vi "fsk_test3_rx.vi"(0 "passband waveform (complex)":T1={"t0"=0.0, "dt"=1.0, "Y"=[]} {"Y" format="%.3f"; "dt" format="%^.2e"; "t0" format="%.4f"}, 1 "FSK system parameters":T2={"samples per symbol (16)"=16, "symbol map"=[], "symbol phase continuity"=enum."continuous"} {"symbol map" format="%.2f"}, 2 "VCO carrier frequency (Hz)":dbl, 3 "passband bandwidth (Hz)":dbl format="%.2p", 4 "reset? (F)":bool, 5 "error in (no error)":errorcluster, 6 "expected sync location (symbols)":i32=-1, 7 "pulse shaping filter coefficients":dbl[](array[numeric]) format="%.2f", 8 "sync location uncertainty (symbols)":i32=10, 9 "matched filter coefficients":dbl[](array[numeric]) format="%.2f", 11 "sync bits":i8[](array[numeric]), 13 "Key Bit Sequence":u32[](array[numeric])) -> (14 "recovered bit sequence":i8[](array[numeric]), 15 "BER":dbl, 16 "recovered complex waveform":T1 {"Y" format="%.3f"; "dt" format="%^.2e"; "t0" format="%.4f"}, 19 "error out":errorcluster)   [LabVIEW 2012]
uses:
  <vilib>/addons/Modulation/Analog/controls/Complex Data Waveform.ctl
  <vilib>/addons/Modulation/Analog/MT Baseband PLL.vi
  <vilib>/addons/Modulation/Analog/MT Downconvert Passband (Complex).vi
  <vilib>/addons/Modulation/Digital/General/MT Generate FSK Synchronization Parameters (bit array).vi
  <vilib>/addons/Modulation/niAMT.lvlib
  <vilib>/addons/Modulation/niDMT.lvlib
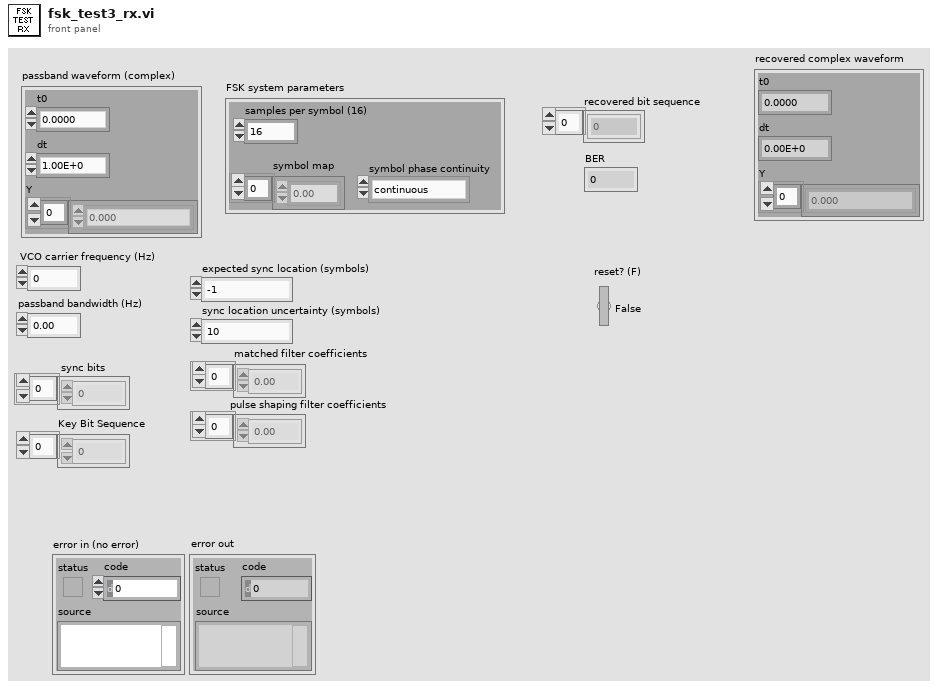
[diagram p1: front panel]
types:
  T1 = typedef "niAMT.lvlib/Complex Data Waveform.ctl" = cluster{"t0":dbl, "dt":dbl, "Y":cdb[]}
  T2 = cluster{"samples per symbol (16)":i32, "symbol map":dbl[], "symbol phase continuity":enum16{"continuous", "discontinuous"}}
  T3 = cluster{"expected sync location (symbols)":i32, "sync sequence":cdb[], "sync location uncertainty (symbols)":i32, "sync indent (symbols)":i32}
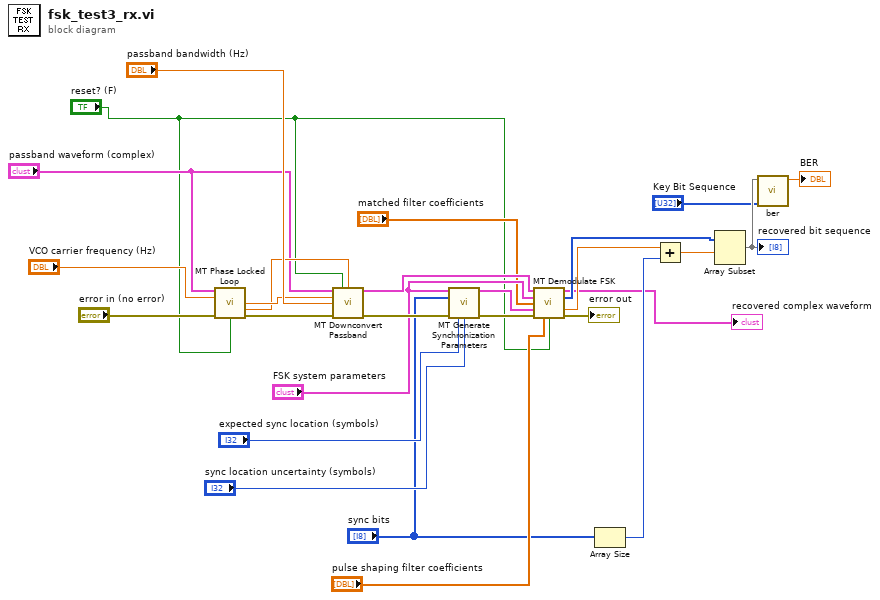
[diagram p0: block diagram]
diagram:
  n1 = call-poly <vilib>:"MT Phase Locked Loop.vi"("baseband waveform (complex)"="passband waveform (complex)", "VCO carrier frequency (Hz)"="VCO carrier frequency (Hz)", "error in (no error)"="error in (no error)", "reset ?(T)"="reset? (F)") -> ("estimated carrier frequency (Hz)"=w24:dbl, "estimated initial phase (degrees)"=w22:dbl, "error out"=w23:errorcluster)  [unwired: 7 in, 2 out]
  n2 = call-poly <vilib>:"MT Downconvert Passband.vi"("complex waveform"="passband waveform (complex)", "reset? (F)"="reset? (F)", "initial phase (deg)"=w22, "carrier frequency (Hz)"=w24, "passband bandwidth (Hz)"="passband bandwidth (Hz)", "error in (no error)"=w23) -> ("downconverted waveform (complex)"=w15:T1, "error out"=w20:errorcluster)  [unwired: 6 in, 2 out]
  n3 = call-poly <vilib>:"MT Generate Synchronization Parameters.vi"("FSK system parameters"="FSK system parameters", "sync bits"="sync bits", "error in (no error)"=w20, "expected sync location (symbols)"="expected sync location (symbols)", "sync location uncertainty (symbols)"="sync location uncertainty (symbols)") -> ("FSK synchronization parameters"=w17:T3, "error out"=w14:errorcluster)  [unwired: 9 in]
  n4 = call <vilib>:"MT Demodulate FSK.vi"("input complex waveform"=w15, "FSK system parameters"="FSK system parameters", "matched filter coefficients"="matched filter coefficients", "synchronization parameters"=w17, "error in (no error)"=w14, "pulse shaping filter coefficients"="pulse shaping filter coefficients", "reset? (T)"="reset? (F)") -> ("recovered complex waveform"=→"recovered complex waveform":T1, "output bit stream"=w11:i8[], "sync found index (symbols)"=w8:dbl, "error out"=→"error out":errorcluster)  [unwired: 4 in, 1 out]
  n5 = Array Size(array="sync bits") -> (size(s)=w9:i32)
  n6 = Add(x=w8, y=w9) -> (x+y=w7:dbl)
  n7 = Array Subset(array=w11, index=w7) -> (w6:i8[])  [unwired: 1 in]
  "recovered bit sequence" <- w6
  n8 = call "ber.vi"("Key Bit Sequence"="Key Bit Sequence", "Recovered Bit Sequence"=w6) -> ("BER"=→"BER":dbl)  [unwired: 9 in]
